vi "_range_table_coerce_double.vi"(7 "Attribute":T1={"Identifier"="", "Descriptive Name"="", "Data Type"=enum."Integer 32", "Command"="", "Access"=enum."Read/Write", "Range Table"="", "Read Callback"="", "Write Callback"="", "Supported Models"="", "Instrument Options"="", "Index"=0, "OPC Wait"=FALSE, "No Status Check"=FALSE, "Cache Only"=FALSE}, 8 "error in":errorcluster caption="error in (no error)", 10 "Double in":dbl, 11 "VISA resource name":refnum<visa-resource-name>) -> (0 "error out":errorcluster, 2 "Double out":dbl, 3 "VISA resource name out":refnum<visa-resource-name>)   [LabVIEW 2022 SP3, in "hmp4000_rsidr_core.lvlib"]
uses:
  hmp4000_rsidr_core.lvlib
  type_Attribute.ctl
  type_Attribute_Data_Type.ctl
  type_ReadWriteAccess.ctl
  _type_Operation_Fgv_RangeTable.ctl
  type_Error_Codes.ctl
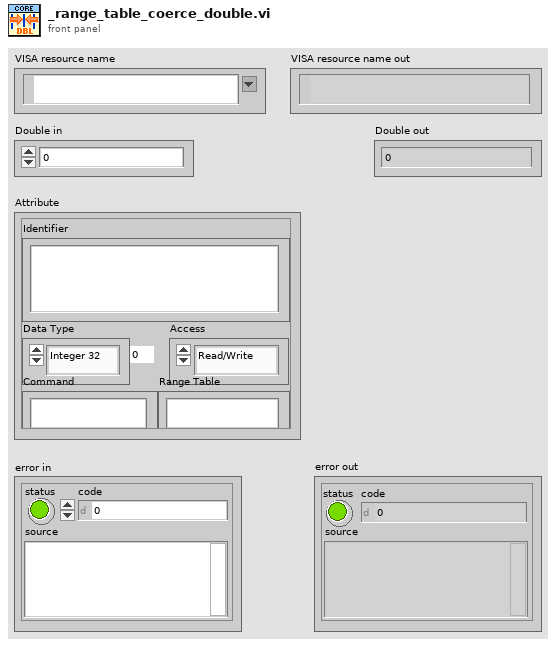
[diagram p1: front panel]
types:
  T1 = typedef "hmp4000_rsidr_core.lvlib/type_Attribute.ctl" = cluster{"Identifier":string, "Descriptive Name":string, "Data Type":T2, "Command":string, "Access":T3, "Range Table":string, "Read Callback":string, "Write Callback":string, "Supported Models":string, "Instrument Options":string, "Index":i32, "OPC Wait":bool, "No Status Check":bool, "Cache Only":bool}
  T2 = typedef "hmp4000_rsidr_core.lvlib/type_Attribute_Data_Type.ctl" = enum16{"Integer 32", "Double", "String", "Boolean", "None", "Integer 64", "RawString"}
  T3 = typedef "hmp4000_rsidr_core.lvlib/type_ReadWriteAccess.ctl" = enum16{"Read Only", "Write Only", "Read/Write"}
  T4 = typedef "hmp4000_rsidr_core.lvlib/_type_Operation_Fgv_RangeTable.ctl" = enum16{"Initialize", "Check", "Coerce", "Get Command String", "Get Numeric Value", "Get Default Value", "Get Range Table Type"}
  T5 = typedef "hmp4000_rsidr_core.lvlib/type_Error_Codes.ctl" = enum16{"No_error", "VISA_err_ResourceNotFound", "VISA_err_Timeout", "VISA_warn_MoreDataAvailable", "RS_err_MissingCallback", "RS_err_InvalidAttribute", "RS_err_InvalidValue", "RS_err_UnknownResource", "RS_err_AlreadyInitialized", "RS_err_InstrumentStatus", "RS_err_BadRepCapName", "RS_err_TypesMismatch", "RS_err_ValueNotSupported", "RS_err_InvalidRngTable", "RS_err_IDqueryFail", "RS_err_UnexpResponse", "VISA_warn_ConfigNotLoaded", "RS_err_AttributeNotReadable", "RS_err_AttributeNotWritable", "RS_err_InstrumentType", "RS_err_InstrumentOption", "VISA_err_InvalidSize", "RS_err_ReliabilityIndicator", "VISA_warn_UnknownStatus", "VISA_warn_TermCharRead", "VISA_err_IO_error", "RS_err_FunctionNotSupported", "VISA_warn_QueueEmpty"}
  T6 = typedef "hmp4000_rsidr_core.lvlib/type_Session_Data.ctl" = cluster{"IDN string":string, "Instrument FW":string, "Instr type":string, "Instr type for err. msg.":string, "Installed Options":string[], "Ignore Error Messages":string, "Logging params":variant, "OPC Timeout":i32, "VISA Timeout":i32, "STB Poll VISA Timeout":i32, "Additional Flags":i32, "Wait Before Read":i32, "Wait Before Write":i32, "Option String Flags":i32, "IO Segment Size":i64, "VISA Access Mode":T7, "Interface Type":T8, "OPC Wait Mode":T9, "Bin Float Number  Format":T10, "Bin Integer Number Format":T11, "Simulate":bool, "VXIcapable":bool, "Duplicate Session":bool, "Add LF to Write":bool, "Logging":bool, "Fast Sweep":bool, "Query Instrument Status":bool, "Check Range":bool, "Check Options":bool}
  T7 = typedef "hmp4000_rsidr_core.lvlib/type_VisaAccessMode.ctl" = u16
  T8 = typedef "hmp4000_rsidr_core.lvlib/type_InterfaceType.ctl" = enum16{"Unknown", "GPIB", "VXI", "GPIB_VXI", "ASRL", "PXI", "TCPIP", "USB", "SOCKET"}
  T9 = typedef "hmp4000_rsidr_core.lvlib/type_OPC_Wait_Mode.ctl" = enum16{"STBpolling", "STBpollingSlow", "STBpollingSuperSlow", "ServiceRequest", "OPCquery"}
  T10 = typedef "hmp4000_rsidr_core.lvlib/type_Binary_Float_Number_Format.ctl" = enum16{"Float_4_Bytes_Swapped", "Float_4_Bytes", "Double_8_Bytes_Swapped", "Double_8_Bytes"}
  T11 = typedef "hmp4000_rsidr_core.lvlib/type_Binary_Integer_Number_Format.ctl" = enum16{"Int32_4_Bytes_Swapped", "Int32_4 Bytes", "Int16_2_Bytes_Swapped", "Int16_2_Bytes"}
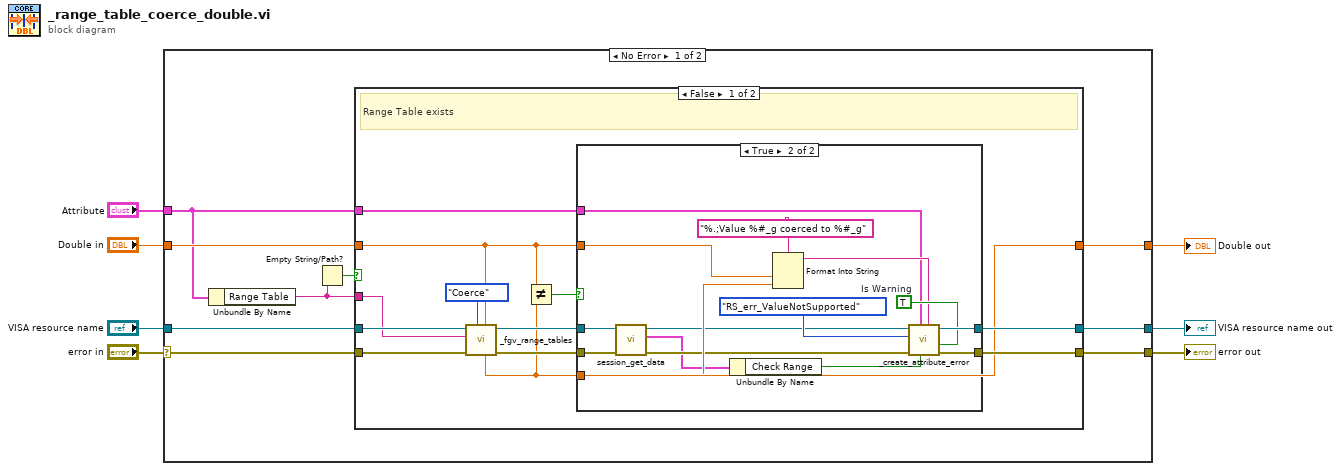
[diagram p0: block diagram]
diagram:
  n1 = case shown="No Error" "error in" {
    selector: "error in" -> [w16 w50]
    tunnel: "VISA resource name" -> [w15 w51]
    tunnel: [w10 w51] -> w7
    tunnel: [w11 w50] -> w6
    tunnel: "Attribute" -> [w8 _]
    tunnel: "Double in" -> [w12 w49]
    tunnel: [w9 w49] -> w1
    frame No Error {
      n2 = Unbundle By Name(w8) -> ("Range Table"=w13:string)
      n3 = Empty String/Path?(string/path=w13) -> (empty?=w14:bool)
      n4 = case shown="False" w14 {
        tunnel: w16 -> [w28 w48]
        tunnel: w15 -> [w27 w47]
        tunnel: w13 -> [w25 _]
        tunnel: w12 -> [w20 w46]
        tunnel: [w22 w48] -> w11
        tunnel: [w21 w47] -> w10
        tunnel: [w18 w46] -> w9
        tunnel: w8 -> [w17 _]
        frame False {
          # "Range Table exists"
          n5 = call "_fgv_range_tables.vi"("Numeric Value in (0.0)"=w20, "Operation"=_type_Operation_Fgv_RangeTable."Coerce", "error in"=w28, "Range Table ID in"=w25, "VISA resource name"=w27) -> ("error out"=w24:errorcluster, "VISA resource name out"=w23:refnum<visa-resource-name>, "Numeric Value out"=w18:dbl)  [unwired: 2 in, 2 out]
          n6 = Not Equal?(x=w20, y=w18) -> (x != y?=w19:bool)
          n7 = case shown="True" w19 {
            tunnel: w20 -> [_ w44]
            tunnel: w24 -> [w30 w36]
            tunnel: w23 -> [w29 w35]
            tunnel: [w30 w42] -> w22
            tunnel: [w29 w41] -> w21
            tunnel: w18 -> [_ w43]
            tunnel: w17 -> [_ w37]
            frame False {
            }
            frame True {
              w40 = TRUE  # Is Warning
              n8 = call "session_get_data.vi"("error in"=w36, "VISA resource name"=w35) -> ("error out"=w34:errorcluster, "Session User Data out"=w32:T6, "VISA resource name out"=w33:refnum<visa-resource-name>)  [unwired: 6 in, 1 out]
              n9 = Unbundle By Name(w32) -> ("Check Range"=w31:bool)
              n10 = Format Into String(format string="%.;Value %#_g coerced to %#_g" ("string"), w44, w43) -> (resulting string=w39:string)  [unwired: 2 in, 1 out]
              n11 = call "_create_attribute_error.vi"("Is Warning (False)"=w40, "Error Elaboration (\"\")"=w39, "Error creation enabled (T)"=w31, "Attribute"=w37, "error in"=w34, "Error Enum in"=type_Error_Codes."RS_err_ValueNotSupported", "VISA resource name"=w33) -> ("error out"=w42:errorcluster, "VISA resource name out"=w41:refnum<visa-resource-name>)  [unwired: 3 in]
            }
          }
        }
        frame True {
          # "No Range Table"
        }
      }
    }
    frame Error {
    }
  }
  "error out" <- w6
  "VISA resource name out" <- w7
  "Double out" <- w1
